vi "FPGA-AI.vi"() -> ()   [LabVIEW 2020]
uses:
  <vilib>/rvi/Emulation/niFpgaGetClockAttributes.vi
  <vilib>/rvi/Emulation/niFpgaSctlEmulationGetInTimedLoop.vi
  <vilib>/rvi/Emulation/niFpgaEmulationReportErrorSimple.vi
  <vilib>/rvi/eio/common/nirviEmuTemplateMethod_errors.vi
  <vilib>/rvi/Emulation/niFpgaCriticalErrorInLSC.vi
  <vilib>/eio/EIONode/EIONode.xnode
panel:
  out "AI Voltage":fxp<+/-,27,5>[](array[numeric])
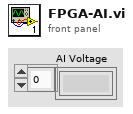
[diagram p1: front panel]
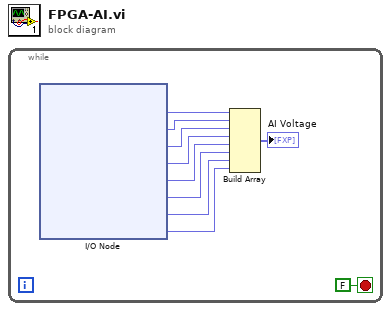
[diagram p0: block diagram]
diagram:
  n1 = while {
    stop <- FALSE stop-if-true
    n2 = xnode "I/O Node"() -> ("Connector0/AI0"=w10:fxp<+/-,27,5>, "Connector0/AI1"=w9:fxp<+/-,27,5>, "Connector0/AI2"=w8:fxp<+/-,27,5>, "Connector0/AI3"=w7:fxp<+/-,27,5>, "Connector0/AI4"=w6:fxp<+/-,27,5>, "Connector0/AI5"=w5:fxp<+/-,27,5>, "Connector0/AI6"=w4:fxp<+/-,27,5>, "Connector0/AI7"=w3:fxp<+/-,27,5>)  [unwired: 8 in, 8 out]
    n3 = Build Array(w10, w9, w8, w7, w6, w5, w4, w3) -> (→"AI Voltage":fxp<+/-,27,5>[])
  }
